vi "Initiate.vi"   [LabVIEW 2014, in "Agilent 34401.lvlib"]
doc: "This low level VI initiates a measurement.\n\n<B>Note:</B>\n\nThis VI has been obsoleted from the driver and is included for compatibility with existing applications. New applications should use the <B>Initiate Measurement VI</B>."
uses:
  <instrlib>/Agilent 34401/Agilent 34401.lvlib
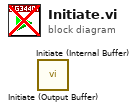
[diagram p0: block diagram]
diagram:
  n1 = call <instrlib>:"Initiate (Output Buffer).vi"() -> ()  [unwired: 10 in, 2 out]
  n2 = call <instrlib>:"Initiate (Internal Buffer).vi"() -> ()  [unwired: 10 in, 2 out]
